vi "Init.vi"(7 "Is Sync":bool) -> (3 "TEMPLATE Msg out":refnum<class "TEMPLATE Msg.lvclass">)   [LabVIEW 2021, in "_Template.lvlib" / "Templates.lvlib" / "TEMPLATE Msg.lvlib" / "TEMPLATE Msg.lvclass"]
uses:
  TEMPLATE Msg.lvclass
  jettl/jettl/Sender/Sender.lvlib
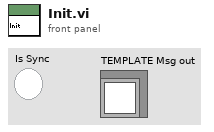
[diagram p1: front panel]
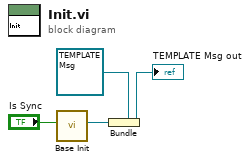
[diagram p0: block diagram]
diagram:
  n1 = call "Base Init.vi"("Is Sync"="Is Sync") -> ("Sender"=w2:refnum<class "Sender.lvclass">)  [unwired: 10 in]
  n2 = Bundle "Bundle"(cluster=refnum<class "TEMPLATE Msg.lvclass"> refnum ("TEMPLATE Msg Strategy out"), w2) -> (→"TEMPLATE Msg out":refnum<class "TEMPLATE Msg.lvclass">)
